vi "RetrieveParameters.vi"(8 "error in (no error)":errorcluster, 11 "ADOParameter in":refnum<class "ADOParameter.lvclass">) -> (0 "error out":errorcluster, 1 "Values":variant[](array[variant]), 2 "Names":string[](array[string]), 3 "ADOParameter out":refnum<class "ADOParameter.lvclass">, 4 "Options":T1(array[cluster]))   [LabVIEW 2020, in "ORM_ADONet.lvlib" / "ADOParameter.lvclass"]
uses:
  ADOParameter.lvclass
  C:/Program Files/National Instruments/LabVIEW 2020/vi.lib/Viviota/shared/ORM.lvlibp/ORM/DynamicParameters/DynamicParameters.lvclass
  <vilib>/Viviota/shared/ORM.lvlibp/ORM/DynamicParameters/Read ParameterNames.vi
  <vilib>/Viviota/shared/ORM.lvlibp/ORM/DynamicParameters/Read ParameterOptions.vi
  <vilib>/Viviota/shared/ORM.lvlibp/ORM/DynamicParameters/Read ParameterValues.vi
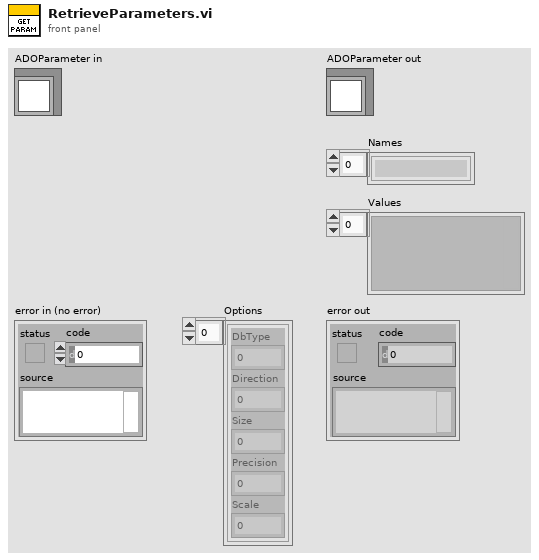
[diagram p1: front panel]
types:
  T1 = cluster{"DbType":i32, "Direction":i32, "Size":i32, "Precision":u8, "Scale":u8}[]
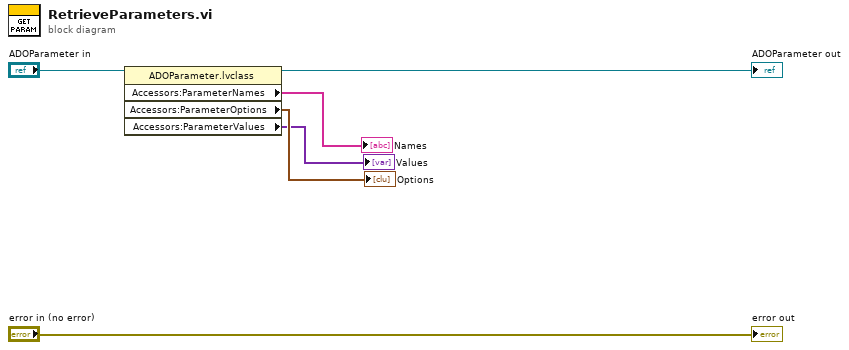
[diagram p0: block diagram]
diagram:
  n1 = property class="ADOParameter.lvclass"(reference="ADOParameter in") -> (reference out=→"ADOParameter out":refnum<class "ADOParameter.lvclass">, "Accessors:ParameterNames"=→"Names":string[], "Accessors:ParameterOptions"=→"Options":T1, "Accessors:ParameterValues"=→"Values":variant[])  [unwired: 1 in, 1 out]
  "error out" <- "error in (no error)"
